vi "04-09 listen to Arduino messages via com port.vi"() -> ()   [LabVIEW 2020]
uses:
  <vilib>/Instr/_visa.llb/VISA Configure Serial Port (Instr).vi
panel:
  out "error out":errorcluster
  in  "data bits (8)":u16=8 min=5 max=8 step=1
  in  "baud rate (9600)":u32=9600
  in  "VISA resource name":refnum<visa-resource-name>
  in  "read count":u32
  out "Array":string[](array[string])
  out "current read buffer":string
  in  "stop":bool
  # "Working off of this example: \nhttps://microcontrollerslab.com/arduino-labview-data-serial-communication/"
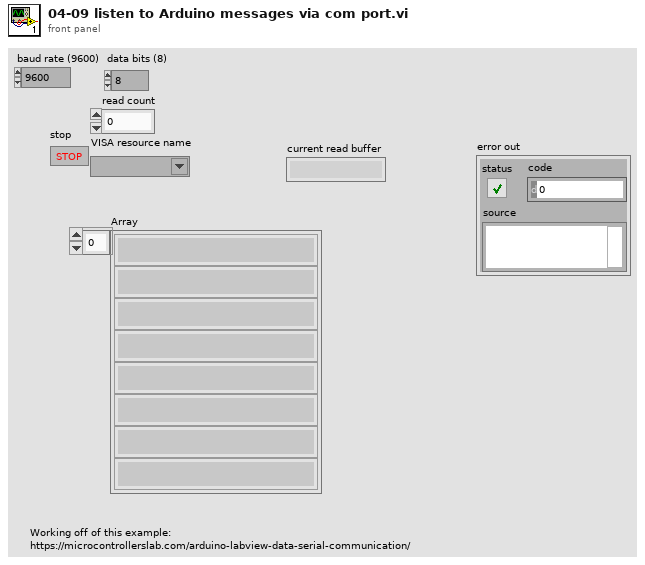
[diagram p1: front panel]
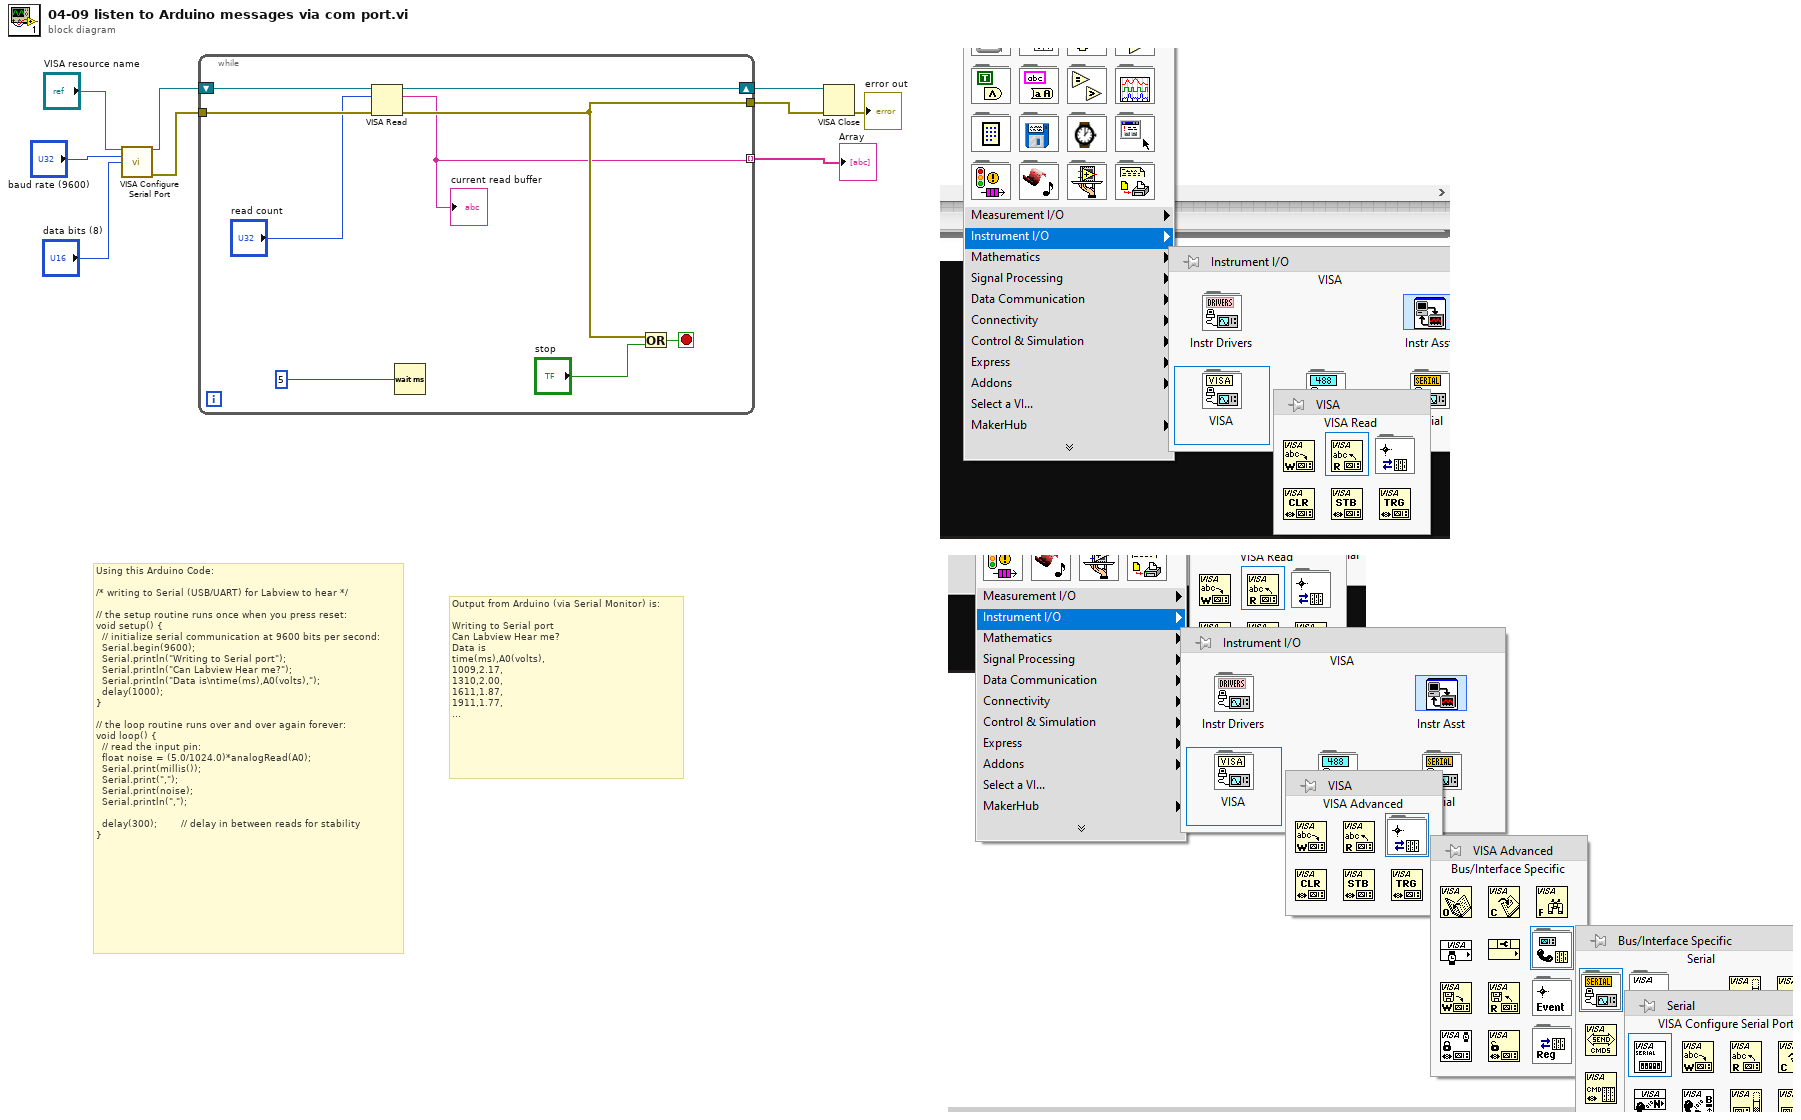
[diagram p0: block diagram]
diagram:
  # "Output from Arduino (via Serial Monitor) is:\n\nWriting to Serial port\nCan Labview Hear me?\nData is\ntime(ms),A0(volts),\n1009,2.17,\n1310,2.00,\n1611,1.87,\n1911,1.77,\n..."
  # "Using this Arduino Code:\n\n/* writing to Serial (USB/UART) for Labview to hear */\n\n// the setup routine runs once when you press reset:\nvoid setup() {\n  // initialize serial communication at 9600 bits per second:\n  Serial.begin(9600);\n  Serial.println(\"Writing to Serial port\");\n  Serial.println(\"Can Labview Hear me?\");\n  Serial.println(\"Data is\\ntime(ms),A0(volts),\");\n  delay(1000);\n}\n\n// the loop routine runs over and over again forever:\nvoid loop() {\n  // read the input pin:\n  float noise = (5.0/1024.0)*analogRead(A0);\n  Serial.print(millis());\n  Serial.print(\",\");\n  Serial.print(noise);\n  Serial.println(\",\");\n  \n  delay(300);        // delay in between reads for stability\n}"
  n1 = call-poly "VISA Configure Serial Port"("VISA resource name"="VISA resource name", "baud rate (9600)"="baud rate (9600)", "data bits (8)"="data bits (8)") -> ("VISA resource name out"=w6:refnum<visa-resource-name>, "error out"=w5:errorcluster)  [unwired: 11 in]
  n2 = while {
    tunnel: [w13] -> w9
    tunnel: w5 -> [w17]
    shift-right: [w16] -> w8
    shift-left: w6 -> [w18]
    tunnel: [w10] -> w7 mode=indexing
    stop <- w14 stop-if-true
    n3 = VISA Read(VISA resource name=w18, byte count="read count", error in (no error)=w17) -> (VISA resource name out=w16:refnum<visa-resource-name>, read buffer=w10:string, error out=w13:errorcluster)  [unwired: 1 out]
    "current read buffer" <- w10
    n4 = Wait (ms)(milliseconds to wait=u32 5) -> ()  [unwired: 1 out]
    n5 = Or(x=w13, y="stop") -> (x .or. y?=w14:bool)
  }
  "Array" <- w7
  n6 = VISA Close(VISA resource name=w8, error in (no error)=w9) -> (error out=→"error out":errorcluster)
